vi "DHE_BuildRootname.vi"(5 "orig rootname":string, 6 "froot":string, 7 "sufix":string, 8 "prefix":string, 9 "basename":string, 10 "imdir":string) -> (1 "rootpath":path, 2 "rootname":string, 3 "basename out":string)   [LabVIEW 2016]
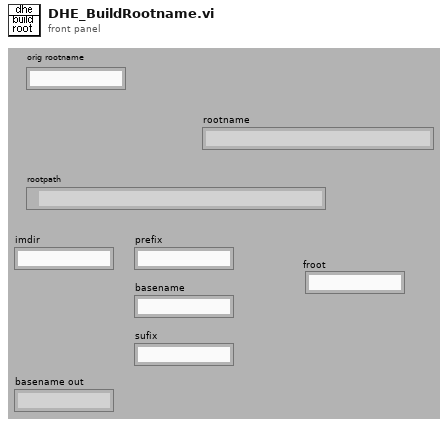
[diagram p1: front panel]
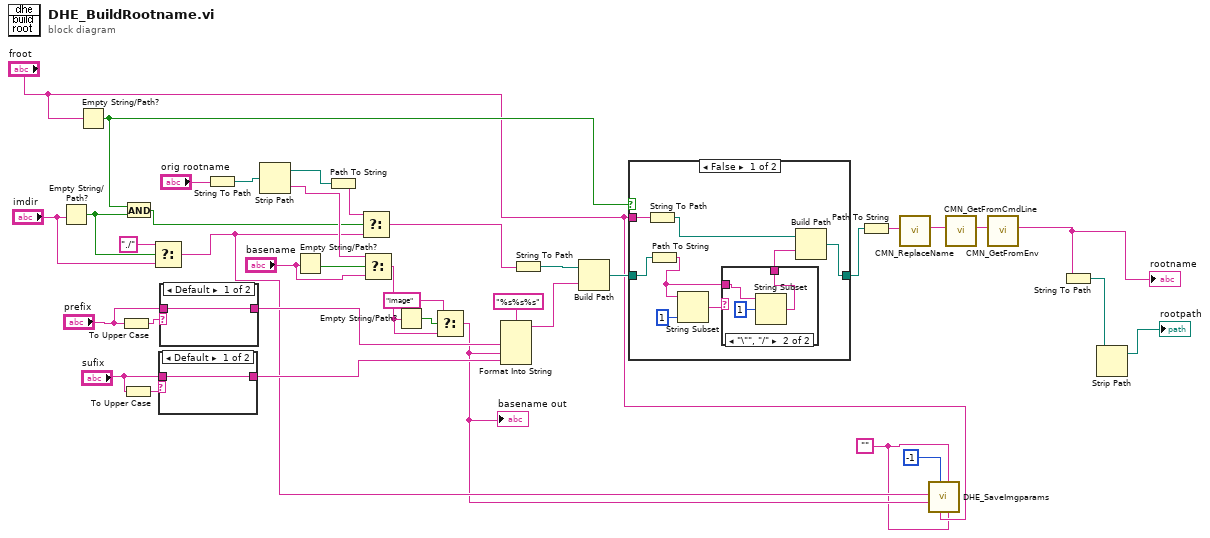
[diagram p0: block diagram]
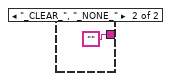
[diagram p4: hidden frame]
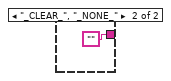
[diagram p5: hidden frame]
diagram:
  w7 = ""
  n1 = Empty String/Path?(string/path="imdir") -> (empty?=w14:bool)
  n2 = Empty String/Path?(string/path="froot") -> (empty?=w16:bool)
  n3 = To Upper Case(1:"prefix") -> (0:w35:string)
  n4 = To Upper Case(1:"sufix") -> (0:w32:string)
  n5 = And(x=w16, y=w14) -> (x .and. y?=w15:bool)
  n6 = Select(t="./", s=w14, f="imdir") -> (s? t:f=w10:string)
  n7 = case shown="Default" w32 {
    tunnel: [w39 ""] -> w31
    tunnel: "sufix" -> [w39 _]
    frame Default {
    }
    frame "_CLEAR_", "_NONE_" {
    }
  }
  n8 = case shown="Default" w35 {
    tunnel: [w41 ""] -> w36
    tunnel: "prefix" -> [w41 _]
    frame Default {
    }
    frame "_CLEAR_", "_NONE_" {
    }
  }
  n9 = String To Path(string="orig rootname") -> (path=w18:path)
  n10 = Strip Path(path=w18) -> (stripped path=w30:path, name=w27:string)
  n11 = Empty String/Path?(string/path="basename") -> (empty?=w29:bool)
  n12 = Path To String(path=w30) -> (string=w28:string)
  n13 = Select(t=w28, s=w15, f=w10) -> (s? t:f=w20:string)
  n14 = Select(t=w27, s=w29, f="basename") -> (s? t:f=w23:string)
  n15 = Empty String/Path?(string/path=w23) -> (empty?=w24:bool)
  n16 = Select(t="image", s=w24, f=w23) -> (s? t:f=w9:string)
  "basename out" <- w9
  n17 = Format Into String(format string="%s%s%s", w36, w9, w31) -> (resulting string=w37:string)  [unwired: 2 in, 1 out]
  n18 = String To Path(string=w20) -> (path=w21:path)
  n19 = Build Path(base path=w21, name or relative path=w37) -> (appended path=w17:path)
  n20 = case shown="False" w16 {
    tunnel: w17 -> [w46 w55]
    tunnel: [w44 w55] -> w6
    tunnel: "froot" -> [w50 _]
    frame False {
      n21 = String To Path(string=w50) -> (path=w49:path)
      n22 = Path To String(path=w46) -> (string=w43:string)
      n23 = String Subset(string=w43, length (rest)=1 ("length (rest)")) -> (substring=w47:string)  [unwired: 1 out]
      n24 = case shown="\"\\\"\", \"/\"" w47 {
        tunnel: [w51 w52] -> w45
        tunnel: w43 -> [w51 w54]
        frame Default {
        }
        frame "\"", "/" {
          n25 = String Subset(string=w54, offset (0)=1) -> (substring=w52:string)  [unwired: 1 out]
        }
      }
      n26 = Build Path(base path=w49, name or relative path=w45) -> (appended path=w44:path)
    }
    frame True {
    }
  }
  n27 = Path To String(path=w6) -> (string=w4:string)
  n28 = call "CMN_ReplaceName.vi"("name in"=w4) -> ("name out"=w3:string)  [unwired: 1 in, 9 out]
  n29 = call "DHE_SaveImgparams.vi"("prefix"=w7, "sufix"=w7, "froot"="froot", "number"=-1, "basename"=w9, "dir"=w10) -> ()  [unwired: 6 out]
  n30 = call "CMN_GetFromCmdLine.vi"("str in"=w3) -> ("str out"=w2:string)  [unwired: 10 out]
  n31 = call "CMN_GetFromEnv.vi"("str in"=w2) -> ("str out"=w1:string)  [unwired: 10 out]
  "rootname" <- w1
  n32 = String To Path(string=w1) -> (path=w5:path)
  n33 = Strip Path(path=w5) -> (stripped path=→"rootpath":path)  [unwired: 1 out]
